vi "Contour Line_Find Intersected Edges (col) Decide Edge.vi"(9 "|/|? (F)":bool, 10 "index":i32, 11 "col":i32) -> (3 "edge":T1)   [LabVIEW 2017, in "NI_AAL_Geometry.lvlib"]
uses:
  <vilib>/Analysis/NI_AAL_Geometry.lvlib
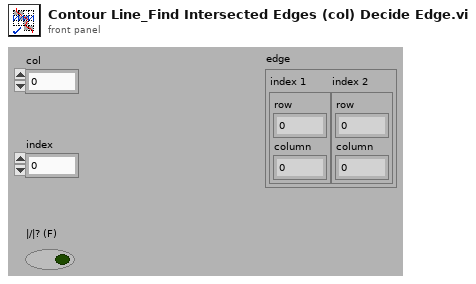
[diagram p1: front panel]
types:
  T1 = cluster{"index 1":cluster{"row":i32, "column":i32}, "index 2":cluster{"row":i32, "column":i32}}
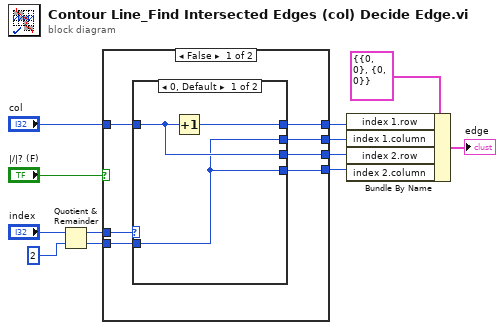
[diagram p0: block diagram]
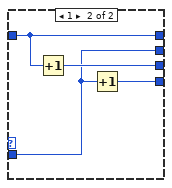
[diagram p2: hidden frame]
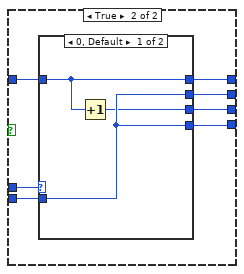
[diagram p3: hidden frame]
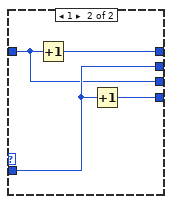
[diagram p4: hidden frame]
diagram:
  n1 = Quotient & Remainder(x="index", y=2) -> (x-y*floor(x/y)=w7:i32, floor(x/y)=w9:i32)
  n2 = case shown="False" "|/|? (F)" {
    tunnel: w9 -> [w15 w28]
    tunnel: w7 -> [w19 w27]
    tunnel: "col" -> [w18 w33]
    tunnel: [w17 w32] -> w5
    tunnel: [w16 w30] -> w4
    tunnel: [w14 w31] -> w3
    tunnel: [w13 w29] -> w2
    frame False {
      n3 = case shown="0, Default" w19 {
        tunnel: w18 -> [w21 w26]
        tunnel: [w22 w26] -> w17
        tunnel: [w21 w25] -> w16
        tunnel: w15 -> [w20 w24]
        tunnel: [w20 w24] -> w14
        tunnel: [w20 w23] -> w13
        frame 0, Default {
          n4 = Increment(x=w21) -> (x+1=w22:i32)
        }
        frame 1 {
          n5 = Increment(x=w26) -> (x+1=w25:i32)
          n6 = Increment(x=w24) -> (x+1=w23:i32)
        }
      }
    }
    frame True {
      n7 = case shown="0, Default" w27 {
        tunnel: w33 -> [w34 w37]
        tunnel: [w34 w38] -> w32
        tunnel: [w35 w37] -> w30
        tunnel: w28 -> [w36 w40]
        tunnel: [w36 w40] -> w31
        tunnel: [w36 w39] -> w29
        frame 0, Default {
          n8 = Increment(x=w34) -> (x+1=w35:i32)
        }
        frame 1 {
          n9 = Increment(x=w37) -> (x+1=w38:i32)
          n10 = Increment(x=w40) -> (x+1=w39:i32)
        }
      }
    }
  }
  n11 = Bundle By Name(cluster=T1 {"index 1"={"row"=0, "column"=0}, "index 2"={"row"=0, "column"=0}} ("intersected edge"), "index 1.row"=w5, "index 1.column"=w3, "index 2.row"=w4, "index 2.column"=w2) -> (→"edge":T1)
